vi "I2C_MASTER_R_W_FINAL.vi"(2 "error in (no error)":errorcluster, 3 "Latch":bool, 4 "y Stepper value":u8, 5 "Arduino mode":T2) -> (0 "error out":errorcluster, 1 "Arduino Data":T1)   [LabVIEW 2018]
uses:
  I2C_MASTER_WRITE_NEW Type Def.ctl
  <vilib>/Studica/Studica Toolkit/Background/I2C Channel.ctl
panel:
  out "Data To Write":u8[](array[numeric])
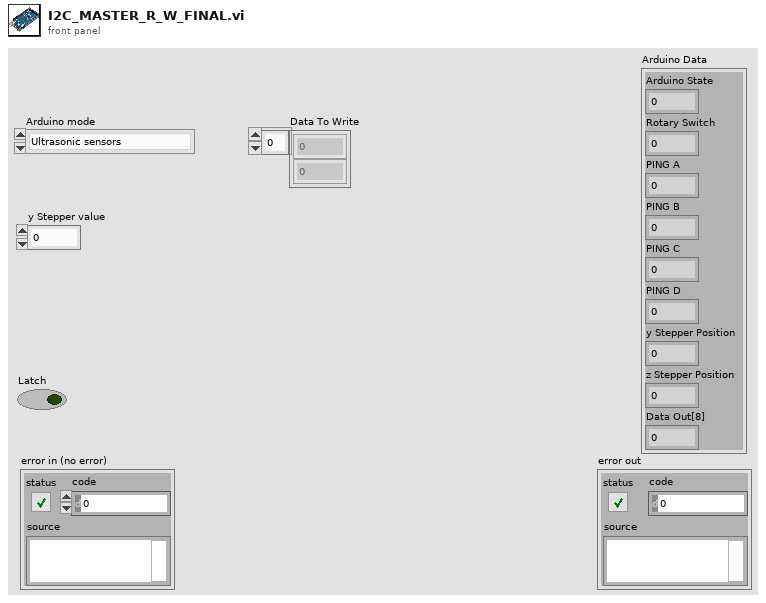
[diagram p1: front panel]
types:
  T1 = cluster{"Arduino State":u8, "Rotary Switch":u8, "PING A":u8, "PING B":u8, "PING C":u8, "PING D":u8, "y Stepper Position":u8, "z Stepper Position":u8, "Data Out[8]":u8}
  T2 = typedef "I2C_MASTER_WRITE_NEW Type Def.ctl" = enum16{"Ultrasonic sensors", "Stepper origin", "zStepper 13.3k", "zStepper 13k", "zStepper 12k", "zStepper 11k", "zStepper 10k", "zStepper 9k", "zStepper 8k", "zStepper 7k", "zStepper 6k", "zStepper 5k", "zStepper 4k", "zStepper 3k", "zStepper 2k", "zStepper 1k", "zStepper 900", "zStepper 800", "zStepper 700", "zStepper 600", "zStepper 500", "zStepper 400", "zStepper 300", "zStepper 200", "zStepper 100", "zStepper 0", "yStepper control", "Open Claw", "Close Claw", "Soft Reset"}
  T3 = typedef "I2C Channel.ctl" = enum16{"Not Connected", "A", "B"}
  T4 = cluster{"I2C Channel":T3, "FPGA VI Reference Out":refnum<k20>}
  T5 = cluster{"Data Out[0]":u8, "Data Out[1]":u8, "Data Out[2]":u8, "Data Out[3]":u8, "Data Out[4]":u8, "Data Out[5]":u8, "Data Out[6]":u8, "Data Out[7]":u8, "Data Out[8]":u8}
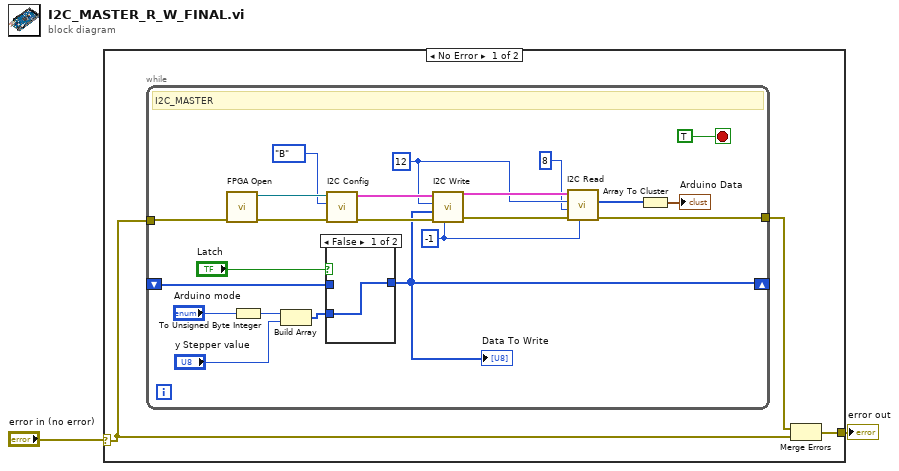
[diagram p0: block diagram]
diagram:
  n1 = case shown="No Error" "error in (no error)" {
    selector: "error in (no error)" -> [w4 w30]
    tunnel: [w5 w30] -> w1
    frame No Error {
      n2 = while {
        tunnel: w4 -> [w21]
        shift-right: [w18] -> _
        shift-left: _ -> [w16]
        tunnel: [w8] -> w3
        stop <- TRUE ("stop") stop-if-true
        w11 = -1 ("Timeout ms (1000)")
        w10 = u8 12 ("Slave Address (7-bit)")
        # "I2C_MASTER"
        n3 = call <vilib>:"FPGA Open.vi"("error in (no error)"=w21) -> ("error out"=w25:errorcluster, "FPGA Reference Out"=w26:refnum<k20>)  [unwired: 9 in]
        n4 = To Unsigned Byte Integer(number="Arduino mode") -> (unsigned 8bit integer=w20:u8)
        n5 = Build Array(w20, "y Stepper value") -> (w19:u8[])
        n6 = case shown="False" "Latch" {
          tunnel: w19 -> [w28 _]
          tunnel: [w28 w29] -> w18
          tunnel: w16 -> [_ w29]
          frame False {
          }
          frame True {
          }
        }
        "Data To Write" <- w18
        n7 = call <vilib>:"I2C Config.vi"("error in (no error)"=w25, "I2C Channel"=I2C_Channel."B", "FPGA Reference"=w26) -> ("error out"=w22:errorcluster, "I2C Ref Out"=w23:T4)  [unwired: 7 in]
        n8 = call <vilib>:"I2C Write.vi"("Timeout ms (1000)"=w11, "error in (no error)"=w22, "Data to Write"=w18, "Slave Address (7-bit)"=w10, "I2C Ref In"=w23) -> ("error out"=w12:errorcluster, "I2C Ref Out"=w13:T4)  [unwired: 5 in]
        n9 = call <vilib>:"I2C Read.vi"("Timeout ms (1000)"=w11, "error in (no error)"=w12, "Bytes to Read"=u32 8, "Slave Address (7-bit)"=w10, "I2C Ref In"=w13) -> ("error out"=w8:errorcluster, "Data Out"=w7:u8[])  [unwired: 4 in, 1 out]
        n10 = Array To Cluster(array=w7) -> (cluster=→"Arduino Data":T5)
      }
      n11 = Merge Errors(w3, w4) -> (w5:errorcluster)
    }
    frame Error {
    }
  }
  "error out" <- w1
